vi "Deadband.vi"(10 "Deadband":dbl, 11 "Robot Velocities":T1) -> (2 "Sending Input?":bool, 3 "Adjusted Robot Velocities":T1)   [LabVIEW 2020]
uses:
  Robot Velocities.ctl
  <vilib>/Analysis/_algsub.llb/Real Vector Norm.vi
  <vilib>/Analysis/NI_AALPro.lvlib
panel:
  in  "New High":dbl
  in  "New Low":dbl
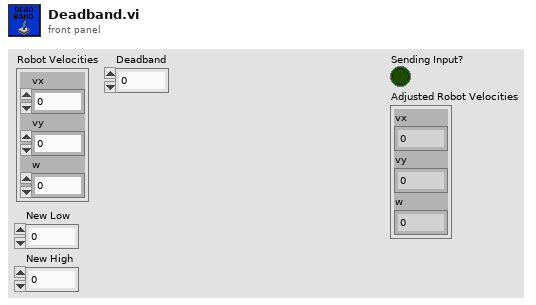
[diagram p1: front panel]
types:
  T1 = typedef "Robot Velocities.ctl" = cluster{"vx":dbl, "vy":dbl, "w":dbl}
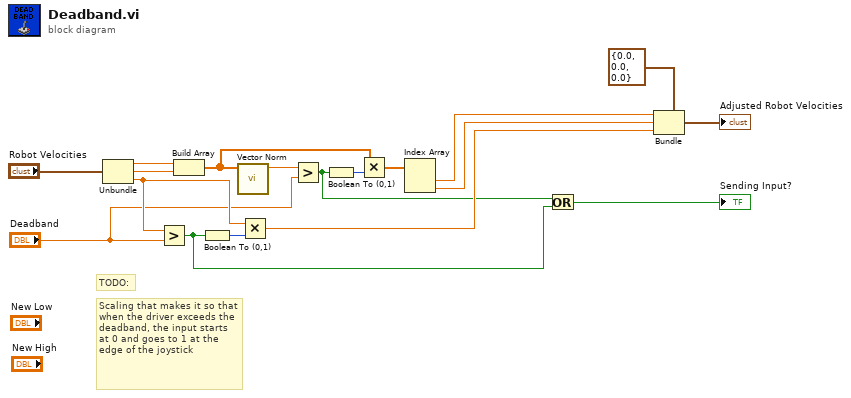
[diagram p0: block diagram]
diagram:
  # "TODO:"
  # "Scaling that makes it so that when the driver exceeds the deadband, the input starts at 0 and goes to 1 at the edge of the joystick"
  n1 = Unbundle("Robot Velocities") -> ("vx"=w17:dbl, "vy"=w16:dbl, "w"=w14:dbl)
  n2 = Greater?(x=w14, y="Deadband") -> (0:w13:bool)
  n3 = Build Array(w17, w16) -> (w8:dbl[])
  n4 = Boolean To (0,1)(Boolean=w13) -> (0, 1=w15:i16)
  n5 = call-poly <vilib>:"Vector Norm.vi"("Input Vector"=w8) -> ("norm"=w10:dbl)  [unwired: 9 in, 1 out]
  n6 = Multiply(x=w14, y=w15) -> (x*y=w3:dbl)
  n7 = Greater?(x=w10, y="Deadband") -> (0:w2:bool)
  n8 = Boolean To (0,1)(Boolean=w2) -> (0, 1=w9:i16)
  n9 = Multiply(x=w8, y=w9) -> (x*y=w6:dbl[])
  n10 = Index Array(array=w6) -> (element #1=w5:dbl, element #2=w4:dbl)  [unwired: 2 in]
  n11 = Or(x=w2, y=w13) -> (x .or. y?=→"Sending Input?":bool)
  n12 = Bundle(cluster=T1 {"vx"=0.0, "vy"=0.0, "w"=0.0} ("Adjusted Robot Velocities"), "vx"=w5, "vy"=w4, "w"=w3) -> (→"Adjusted Robot Velocities":T1)
